vi "Write Outgoing Bytes.vi"(8 "error in (no error)":errorcluster, 10 "Bytes":u8[](array[numeric]) format="%08b", 11 "LocalQueueConnection in":refnum<class "LocalQueueConnection.lvclass">) -> (0 "error out":errorcluster, 3 "LocalQueueConnection":refnum<class "LocalQueueConnection.lvclass">)   [LabVIEW 2013, in "MQTT_Queue.lvlib" / "LocalQueueConnection.lvclass"]
uses:
  LocalQueueConnection.lvclass
  LocalQueueConnection.lvclass/LocalQueueConnection.ctl
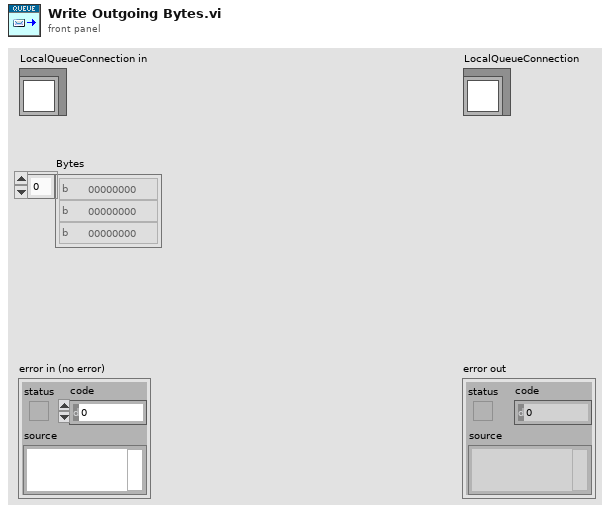
[diagram p1: front panel]
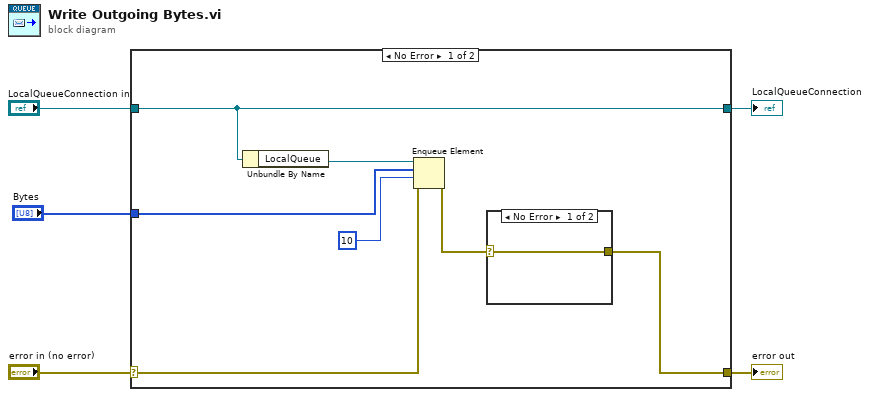
[diagram p0: block diagram]
diagram:
  n1 = case shown="No Error" "error in (no error)" {
    selector: "error in (no error)" -> [w7 w16]
    tunnel: [w11 w16] -> w4
    tunnel: [w12 w15] -> w2
    tunnel: "LocalQueueConnection in" -> [w12 w15]
    tunnel: "Bytes" -> [w9 _]
    frame No Error {
      n2 = Unbundle By Name(w12) -> ("LocalQueue"=w10:refnum<queue>)
      n3 = Enqueue Element(queue=w10, element=w9, timeout in ms (-1)=10 ("timeout ms (25000)"), error in (no error)=w7) -> (error out=w6:errorcluster)  [unwired: 2 out]
      n4 = case shown="No Error" w6 {
        selector: w6 -> [w13 w14]
        tunnel: [w13 w14] -> w11
        frame No Error {
        }
        frame Error {
        }
      }
    }
    frame Error {
    }
  }
  "error out" <- w4
  "LocalQueueConnection" <- w2
